vi "Interlock 32T Net Client Globals.vi"() -> ()   [LabVIEW 2023]
doc: "Author: Scott Hannahs <sth@magnet.fsu.edu>\nCopyright 2018 Florida State University, All rights reserved."
panel:
  in  "User Controls":string[](array[string])=["Setpoint [T]", "Slew rate [T/min]", "PS Action"]
  in  "Admin Controls":string[](array[string])=["Save FPGA Config"]
  in  "Network Read Time Out (mS)":i32=2000
  in  "Connection Time Out (mS)":i32=10000
  in  "Operator Controls":string[](array[string])=["Read FPGA Config", "Clear Quench", "Client Loop Time (mS)", "Reset Battery Alarm"]
  in  "Intitial Controls":string[](array[string])=["Version FPGA", "Version RT System", "Start DateStamp", "Clear Quench"]
  in  "Server Comm Port":u16=17008
  in  "Server Address":string="SCM4-Interlock.ad.magnet.fsu.edu"
  in  "Misc Controls":string[](array[string])=["Save FPGA Config", "Read FPGA Config"]
  in  "Global Controls":string[](array[string])=["Ch Scale", "HTS Shunt Offset (V)", "LTS Shunt Offset (V)", "Crowbar Loop Time (ms)", "Ramp To Zero loop Time (ms)", "WDT Check Loop Ticks", "Trip Threshold Currents", "Contactor Off Current", "Contactor On Current", "Quench Loop Thresh", "SW1 Vout Thresh", "HTS Current Mismatch", "LTS Current Mismatch", "DAQ Loop Timer (Ticks)", "Contactor Closed Time (mS)", "Crowbar Reset Countdown Length (ms)", "Helium Low Level", "# Low Readings", "Battery Low Warn", "Notification Email", "Helium Level #1 VISA Resource", "Helium Level #2 VISA Resource", "LTS Power Supply Control", "HTS Power Supply Control", "Prologix GPIB Address", "LTS DMM GPIB", "HTS DMM GPIB", "Crowbar Unlock Safe Limit", "Logic PWR Thresh", "Batt Mon Wait Timeout", "Batt Mon Read Timeout", "Field Diff Max", "Field Diff Count", "Max combined field"]
  in  "Server Network Ref":refnum<k5>
  in  "Interlock 32T Data Period":dbl=0.0001024
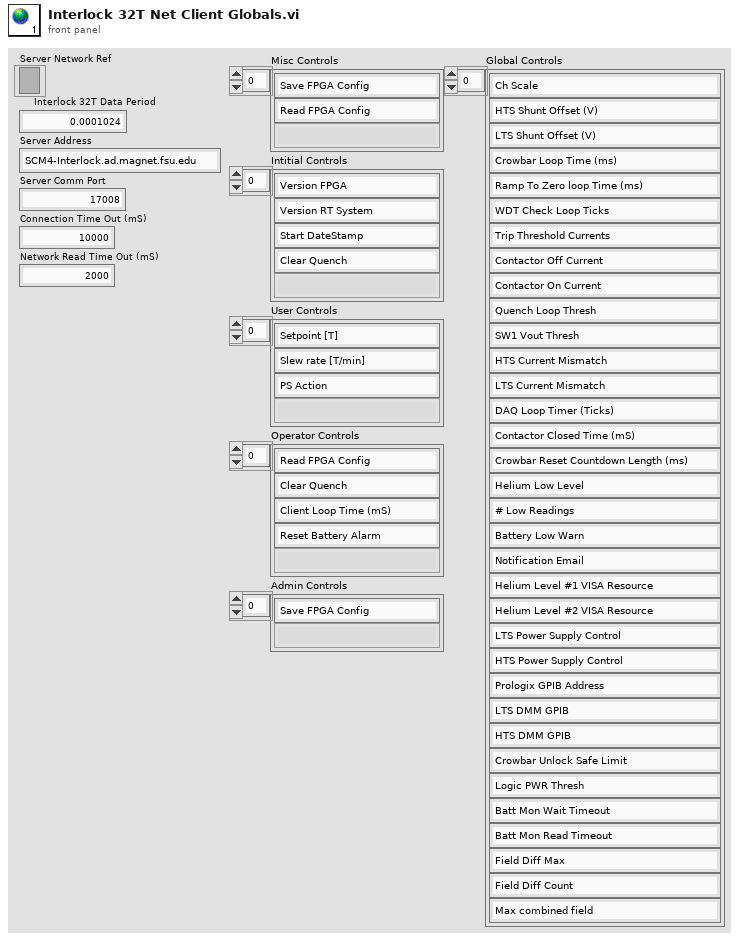
[diagram p1: front panel]
diagram:
